vi "SEA 9811_LegalInformation.vi"   [LabVIEW 2017]
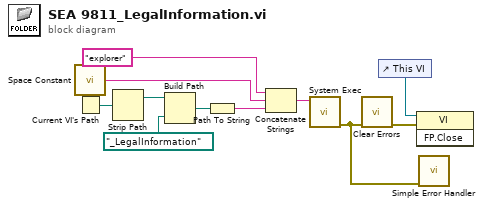
[diagram p0: block diagram]
diagram:
  n1 = call <vilib>:"Space Constant.vi"() -> ("String"=w8:string)
  n2 = Current VI's Path() -> (path=w7:path)
  n3 = Strip Path(path=w7) -> (stripped path=w6:path)  [unwired: 1 out]
  n4 = Build Path(base path=w6, name or relative path=path "_LegalInformation") -> (appended path=w4:path)
  n5 = Path To String(path=w4) -> (string=w11:string)
  n6 = Concatenate Strings("explorer" ("string"), w8, w11) -> (w10:string)
  n7 = call <vilib>:"System Exec.vi"("command line"=w10) -> ("error out"=w2:errorcluster)  [unwired: 7 in, 3 out]
  n8 = call <vilib>:"Clear Errors.vi"("error in (no error)"=w2) -> ("error out"=w1:errorcluster)  [unwired: 5 in, 1 out]
  n9 = control-ref of="This VI"() -> (w3:refnum<vi>)
  n10 = invoke class="VI" method="FP.Close"(reference=w3, error in=w1) -> ()  [unwired: 1 in, 3 out]
  n11 = call <vilib>:"Simple Error Handler.vi"("error in (no error)"=w2) -> ()  [unwired: 4 in, 5 out]
